vi "Configure Control AI Range(DI Scale).vi"(0 "VISA resource name":refnum<visa-resource-name>, 1 "Unit No. (0)":i32 min=0 max=6, 2 "Span":T2={"DI Type (0: LVL)"=0, "Lower Span (0)"=0, "Upper Span (1)"=1} {"DI Type (0: LVL)" items=["LVL", "DI"]; "Upper Span (1)" min=-99999 max=99999 step=1; "Lower Span (0)" min=-99999 max=99999 step=1}, 3 "Scaling":T1={"Floating point position (2)"=2, "Lower Scaling (0)"=0.0, "Upper Scaling (100.00)"=100.0, "Unit Character (\"\")"=""} {"Upper Scaling (100.00)" format="%_6g"; "Lower Scaling (0)" format="%_6g"; "Floating point position (2)" min=0 max=5 step=1}, 4 "Module No.(0)":i32 min=0 max=9, 5 "AI No.(1)":i32=1 min=1 max=2, 7 "error in (no error)":errorcluster) -> (20 "VISA resource name out":refnum<visa-resource-name>, 21 "AI No.":i32, 24 "Unit No.":i32, 25 "Module No.":i32, 27 "error out":errorcluster)   [LabVIEW 2020, in "Yokogawa GX Series.lvlib"]
doc: "Set DI range of AI channel in PID module.\n\nCommand: SCtrlRangeAI"
uses:
  <instrlib>/Yokogawa GX Series/Yokogawa GX Series.lvlib
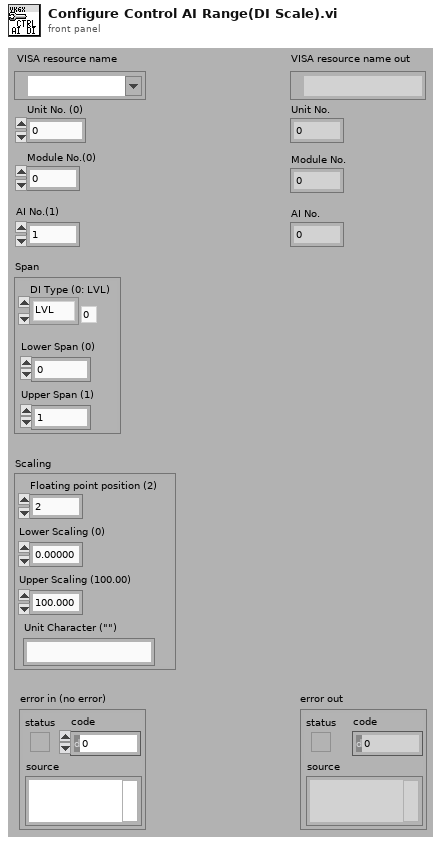
[diagram p1: front panel]
types:
  T1 = cluster{"Floating point position (2)":i32, "Lower Scaling (0)":dbl, "Upper Scaling (100.00)":dbl, "Unit Character (\"\")":string}
  T2 = cluster{"DI Type (0: LVL)":i32, "Lower Span (0)":i32, "Upper Span (1)":i32}
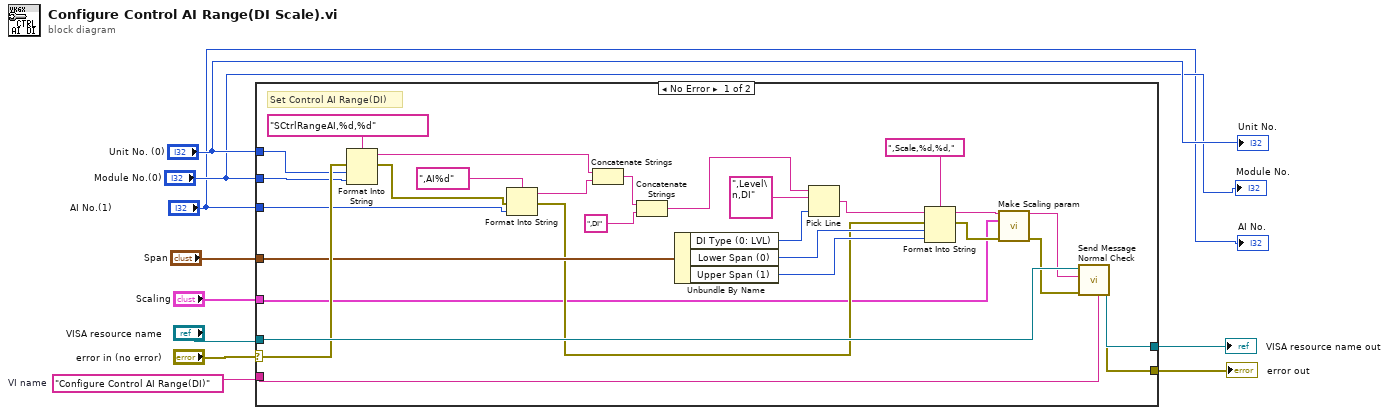
[diagram p0: block diagram]
diagram:
  w6 = "Configure Control AI Range(DI)"  # VI name
  n1 = case shown="No Error" "error in (no error)" {
    selector: "error in (no error)" -> [w35 w40]
    tunnel: [w39 w41] -> w10
    tunnel: [w38 w40] -> w9
    tunnel: "VISA resource name" -> [w37 w41]
    tunnel: w6 -> [w34 _]
    tunnel: "Unit No. (0)" -> [w33 _]
    tunnel: "Module No.(0)" -> [w32 _]
    tunnel: "AI No.(1)" -> [w30 _]
    tunnel: "Span" -> [w18 _]
    tunnel: "Scaling" -> [w13 _]
    frame No Error {
      # "Set Control AI Range(DI)"
      n2 = Format Into String(format string="SCtrlRangeAI,%d,%d", error in=w35, w33, w32) -> (resulting string=w28:string, error out=w29:errorcluster)  [unwired: 1 in]
      n3 = Format Into String(format string=",AI%d", error in=w29, w30) -> (resulting string=w27:string, error out=w17:errorcluster)  [unwired: 1 in]
      n4 = Concatenate Strings(w28, w27) -> (w26:string)
      n5 = Concatenate Strings(w26, ",DI") -> (w19:string)
      n6 = Unbundle By Name(w18) -> ("DI Type (0: LVL)"=w23:i32, "Lower Span (0)"=w21:i32, "Upper Span (1)"=w20:i32)
      n7 = Pick Line(string ("")=w19, multi-line string=",Level\n,DI", line index=w23) -> (output string=w22:string)
      n8 = Format Into String(format string=",Scale,%d,%d,", initial string=w22, error in=w17, w21, w20) -> (resulting string=w15:string, error out=w14:errorcluster)
      n9 = call <instrlib>:"Make Scaling param.vi"("String (\"\")"=w15, "Scaling"=w13, "error in (no error)"=w14) -> ("String After"=w12:string, "error out"=w11:errorcluster)  [unwired: 11 in]
      n10 = call <instrlib>:"Send Message Normal Check.vi"("Source (\"\")"=w34, "error in (no error)"=w11, "Send Message (\"\")"=w12, "VISA resource name"=w37) -> ("error out"=w38:errorcluster, "VISA resource name out"=w39:refnum<visa-resource-name>)  [unwired: 2 in, 4 out]
    }
    frame Error {
    }
  }
  "error out" <- w9
  "VISA resource name out" <- w10
  "Unit No." <- "Unit No. (0)"
  "Module No." <- "Module No.(0)"
  "AI No." <- "AI No.(1)"
